vi "TC_B_VtoC.vi"(11 "Thermocouple Voltage":dbl caption="热电偶电压" format="%0.6f") -> (3 "T(c)":dbl format="%#_16f")   [LabVIEW 2012]
doc: "功能：\n\nB型热电偶电压转换为摄氏度。\n\ncsxcs_366创建。"
uses:
  <vilib>/Analysis/polynomials.llb/Scalar Polynomial Evaluation (DBL).vi
  <vilib>/Analysis/NI_AALPro.lvlib
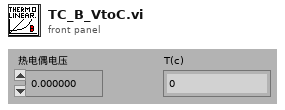
[diagram p1: front panel]
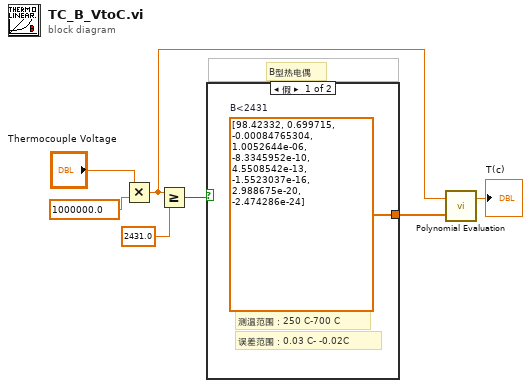
[diagram p0: block diagram]
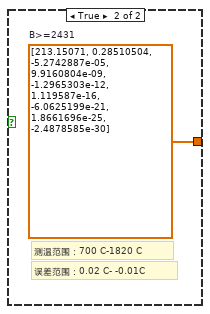
[diagram p2: hidden frame]
diagram:
  # "B型热电偶"
  n1 = Multiply(x="Thermocouple Voltage", y=1000000.0) -> (x*y=w2:dbl)
  n2 = Greater Or Equal?(x=w2, y=2431.0) -> (x >= y?=w4:bool)
  n3 = case shown="假" w4 {
    tunnel: [w8 w9] -> w3
    frame False {
      w8 = dbl[] [98.42332, 0.699715, -0.00084765304, 1.0052644e-06, -8.3345952e-10, 4.5508542e-13, -1.5523037e-16, 2.988675e-20, -2.474286e-24]  # B<2431
      # "误差范围：0.03 C- -0.02C"
      # "测温范围：250 C-700 C"
    }
    frame True {
      w9 = dbl[] [213.15071, 0.28510504, -5.2742887e-05, 9.9160804e-09, -1.2965303e-12, 1.119587e-16, -6.0625199e-21, 1.8661696e-25, -2.4878585e-30]  # B>=2431
      # "误差范围：0.02 C- -0.01C"
      # "测温范围：700 C-1820 C"
    }
  }
  n4 = call-poly <vilib>:"Polynomial Evaluation.vi"("P(x)"=w3, "a"=w2) -> ("P(a)"=→"T(c)":dbl)  [unwired: 1 out]
